vi "Rename.vi"(9 "Replacement String":string=".*", 10 "Split Key":string, 11 "Filenames In":string[](array[string])) -> (3 "Filenames Out":string[](array[string]))   [LabVIEW 2022 SP3]
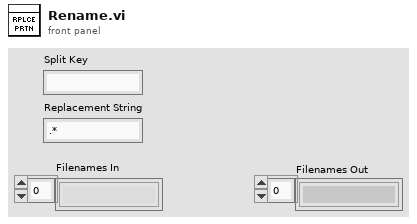
[diagram p1: front panel]
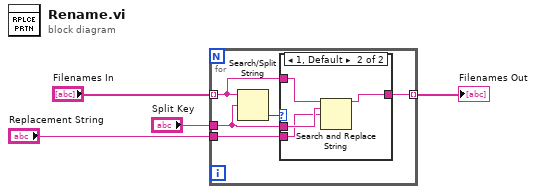
[diagram p0: block diagram]
diagram:
  n1 = for {
    tunnel: "Filenames In" -> [w6] mode=indexing
    tunnel: "Replacement String" -> [w9]
    tunnel: "Split Key" -> [w5]
    tunnel: [w7] -> w2 mode=indexing
    n2 = Search/Split String(string=w6, search string/char (-)=w5) -> (offset of match=w8:i32)  [unwired: 1 in, 2 out]
    n3 = case shown="1, Default" w8 {
      tunnel: w9 -> [_ w12]
      tunnel: [w10 w11] -> w7
      tunnel: w6 -> [w10 w14]
      tunnel: w5 -> [_ w13]
      frame -1 {
      }
      frame 1, Default {
        n4 = Search and Replace String(input string=w14, search string=w13, replace string=w12) -> (result string=w11:string)  [unwired: 5 in, 3 out]
      }
    }
  }
  "Filenames Out" <- w2
